vi "Intake_Test.vi"(11 "Joystick_Out":T1) -> ()   [LabVIEW 2020]
uses:
  Subsystems/Intake/Intake_control_states.ctl
  Subsystems/Intake/Intake_cluster.ctl
  Globals/Intake_Globals.vi
  Utility VIs/Joystick_Controls.ctl
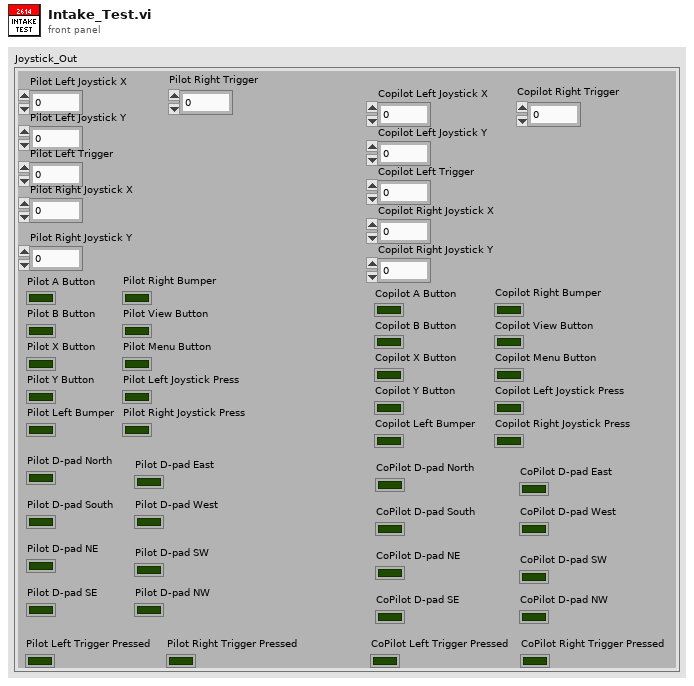
[diagram p1: front panel]
types:
  T1 = typedef "Joystick_Controls.ctl" = cluster{"Pilot Left Joystick X":dbl, "Pilot Left Joystick Y":dbl, "Pilot A Button":bool, "Pilot B Button":bool, "Pilot X Button":bool, "Pilot Y Button":bool, "Pilot Left Bumper":bool, "Pilot Right Bumper":bool, "Pilot View Button":bool, "Pilot Menu Button":bool, "Pilot Left Joystick Press":bool, "Pilot Right Joystick Press":bool, "Pilot Left Trigger":dbl, "Pilot Right Joystick X":dbl, "Pilot Right Joystick Y":dbl, "Pilot Right Trigger":dbl, "Copilot Left Joystick X":dbl, "Copilot Left Joystick Y":dbl, "Copilot A Button":bool, "Copilot B Button":bool, "Copilot X Button":bool, "Copilot Y Button":bool, "Copilot Left Bumper":bool, "Copilot Right Bumper":bool, "Copilot View Button":bool, "Copilot Menu Button":bool, "Copilot Left Joystick Press":bool, "Copilot Right Joystick Press":bool, "Copilot Left Trigger":dbl, "Copilot Right Joystick X":dbl, "Copilot Right Joystick Y":dbl, "Copilot Right Trigger":dbl, "Pilot D-pad North":bool, "Pilot D-pad South":bool, "Pilot D-pad East":bool, "Pilot D-pad West":bool, "Pilot D-pad NE ":bool, "Pilot D-pad SE":bool, "Pilot D-pad SW":bool, "Pilot D-pad NW":bool, "CoPilot D-pad North":bool, "CoPilot D-pad South":bool, "CoPilot D-pad East":bool, "CoPilot D-pad West":bool, "CoPilot D-pad NE":bool, "CoPilot D-pad SE":bool, "CoPilot D-pad SW":bool, "CoPilot D-pad NW":bool, "Pilot Left Trigger Pressed":bool, "Pilot Right Trigger Pressed":bool, "CoPilot Left Trigger Pressed":bool, "CoPilot Right Trigger Pressed":bool}
  T2 = typedef "Intake_cluster.ctl" = cluster{"control_states":T3, "%Vbus":dbl, "Trigger?":bool, "Manual_Extend?":bool, "Auto_Notifier":refnum<notifier>, "Step":dbl, "Parameter 1":dbl, "Parameter 2":dbl, "Parameter 3":dbl}
  T3 = typedef "Intake_control_states.ctl" = enum16{"No_Op", "Intake", "Manual", "Outtake"}
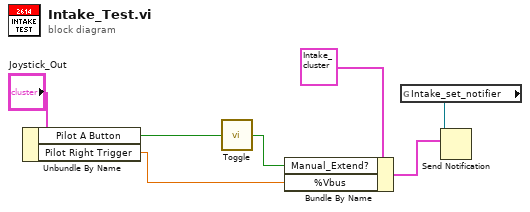
[diagram p0: block diagram]
diagram:
  n1 = Unbundle By Name("Joystick_Out") -> ("Pilot A Button"=w2:bool, "Pilot Right Trigger"=w3:dbl)
  n2 = call "Toggle.vi"("Boolean"=w2) -> ("Boolean Out"=w1:bool)
  n3 = Bundle By Name(cluster=T2 {"control_states"=enum."Intake", "%Vbus"=0.0, "Trigger?"=FALSE, "Manual_Extend?"=FALSE, "Auto_Notifier"=refnum, "Step"=0.0, "Parameter 1"=0.0, "Parameter 2"=0.0, "Parameter 3"=0.0} ("Intake_cluster"), "Manual_Extend?"=w1, "%Vbus"=w3) -> (w6:T2)
  n4 = global read "Intake_Globals.vi" "Intake_set_notifier"() -> (w7:refnum<notifier>)
  n5 = Send Notification(notification=w6, notifier=w7) -> ()  [unwired: 1 in, 2 out]
